vi "DriverCameraWindow.vi"() -> ()   [LabVIEW 2025]
uses:
  DashBoardGlobals.vi
panel:
  out "Camera Perf":string
  in  "Camera Settings":T1={"Frame Rate"=30, "Compression"=30, "Size"=1, "DB Camera Config"=FALSE} {"Frame Rate" scale=1.0..30.0; "Compression" scale=100.0..-1.0; "Size" items=["640x480", "640x360", "320x240", "320x180", "160x120", "160x90"]}
  out "Image Message":string="Timeout in Camera Communications"
  out "Camera Image":T2(plugin-control)
  in  "Camera Name":string(combo)="No Camera Selection"
  # "HW"
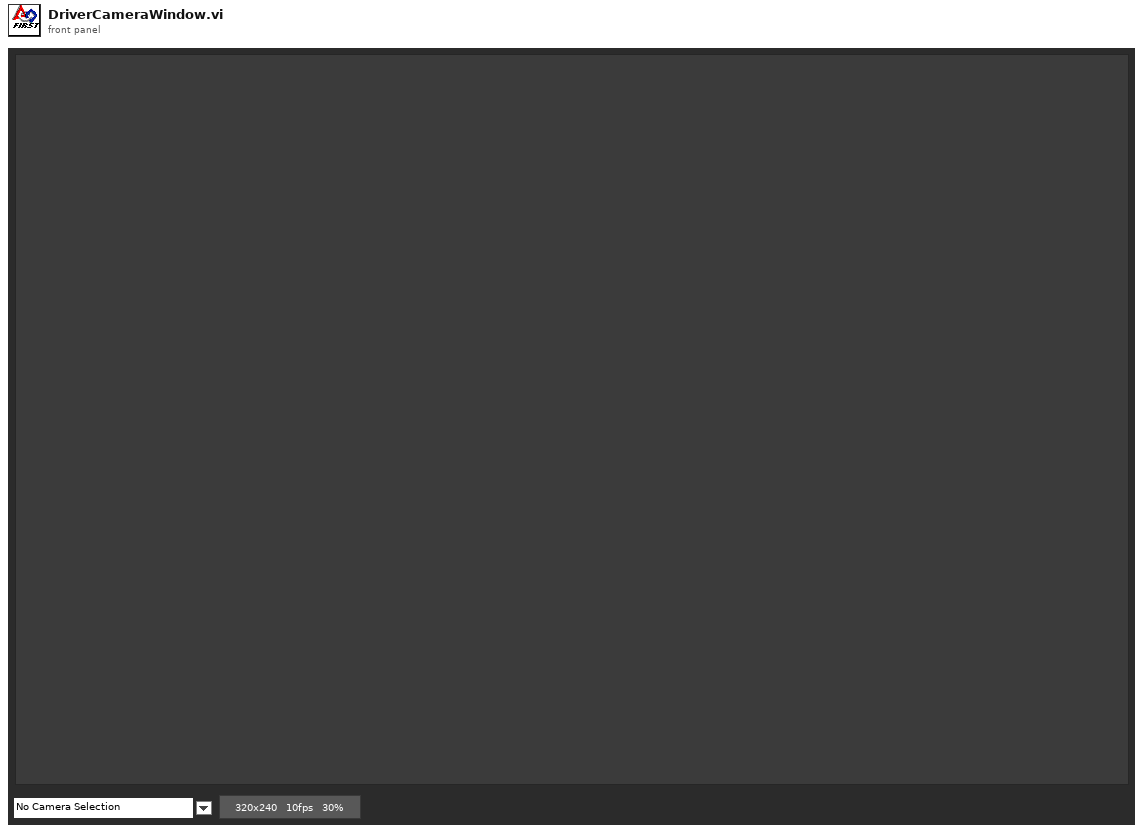
[diagram p1: front panel]
types:
  T1 = cluster{"Frame Rate":i32, "Compression":i32, "Size":u16, "DB Camera Config":bool}
  T2 = typedef "IMAQ Image.ctl" = refnum<image>
  T3 = cluster{"Save Path":path, "Interval (s)":dbl, "Keep":i32}
  T4 = typedef "Image Type" = u32
  T5 = cluster{"Global Rectangle":i32[], "Contours":cluster{"Contour Type":u32, "ROI Type":u32, "Points":i32[]}[]}
  T6 = cluster{"Camera Name":string, string, "Saved DB Images Info":cluster{"Save Path":path, "Interval (s)":dbl, "Keep":i32}}
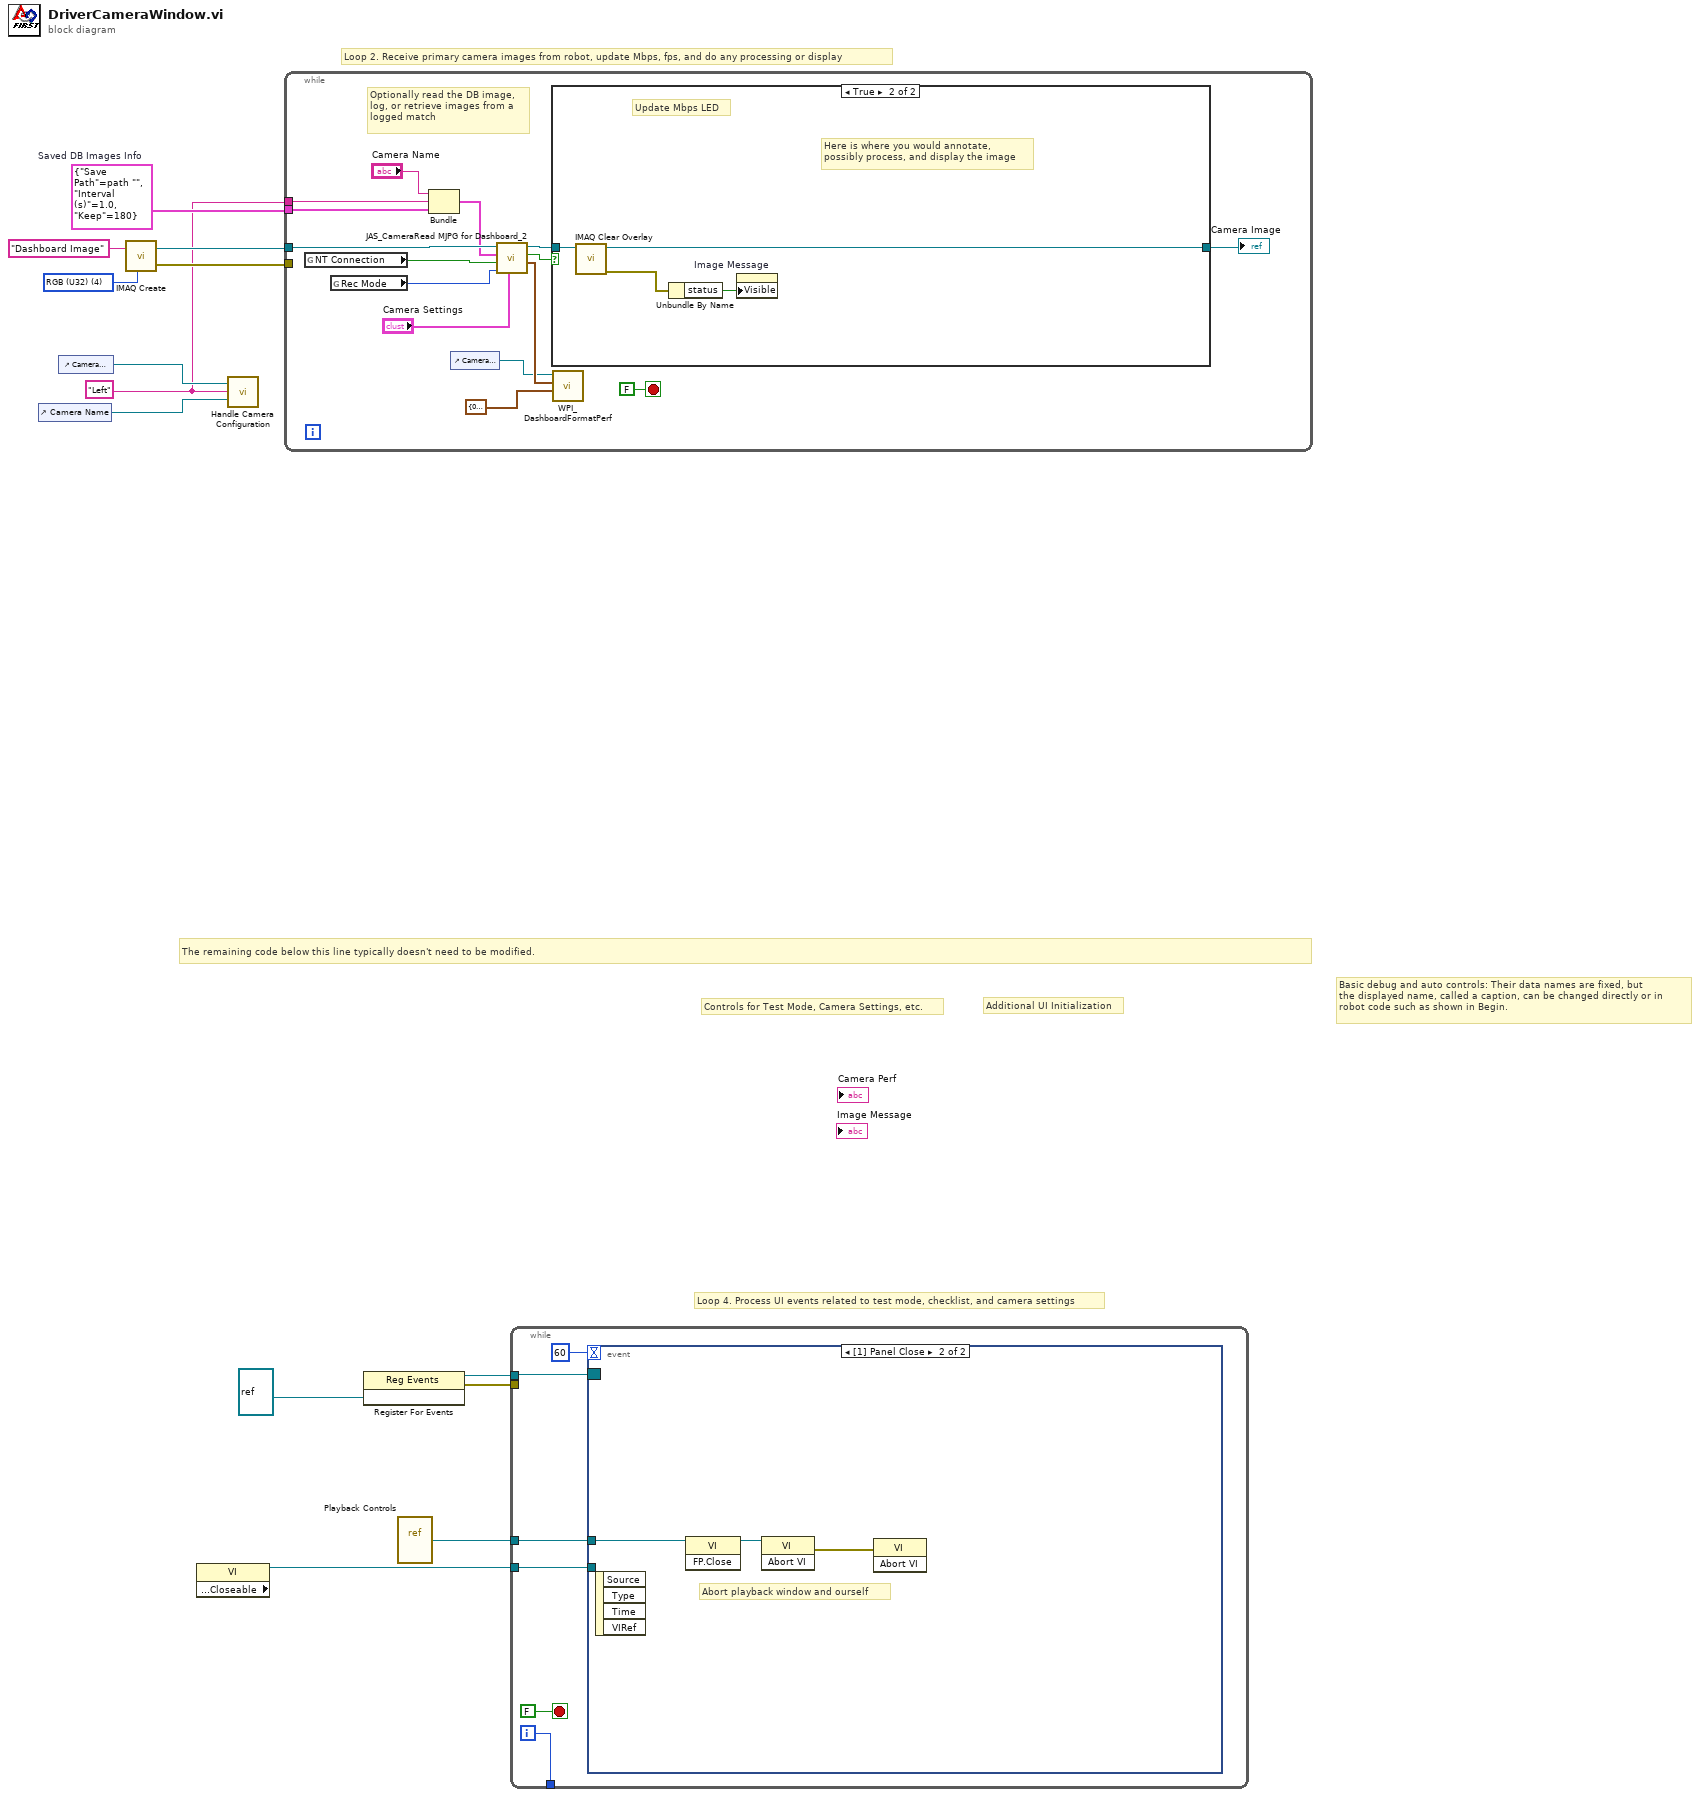
[diagram p0: block diagram]
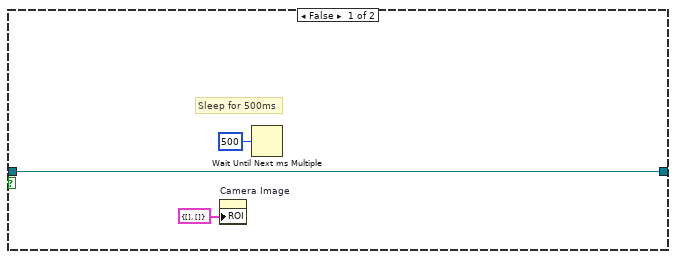
[diagram p2: hidden frame]
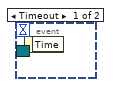
[diagram p3: hidden frame]
diagram:
  w2 = T3 {"Save Path"=path "", "Interval (s)"=1.0, "Keep"=180}  # Saved DB Images Info
  w1 = "Left"
  w13 = T4 4 items=["Grayscale (U8)", "Grayscale (I16)", "Grayscale (SGL)", "Complex (CSG)", "RGB (U32)", "HSL (U32)", "RGB (U64)"] ("Image Type")
  # "Basic debug and auto controls: Their data names are fixed, but\nthe displayed name, called a caption, can be changed directly or in\nrobot code such as shown in Begin."
  # "Controls for Test Mode, Camera Settings, etc."
  # "Additional UI Initialization"
  # "The remaining code below this line typically doesn't need to be modified."
  # "Loop 4. Process UI events related to test mode, checklist, and camera settings"
  # "Loop 2. Receive primary camera images from robot, update Mbps, fps, and do any processing or display"
  n1 = control-ref of="Camera Name"() -> (w3:refnum<vi>)
  n2 = control-ref of="Camera Settings"() -> (w4:refnum<vi>)
  n3 = call "IMAQ Create"("Image Name"="Dashboard Image", "Image Type"=w13) -> ("New Image"=w11:T2, "error out"=w10:errorcluster)  [unwired: 2 in, 1 out]
  n4 = property class="VI" props=["Front Panel.Closeable"]() -> (reference out=w5:refnum<vi>)  [unwired: 2 in, 2 out]
  n5 = call "Handle Camera Configuration.vi"("CameraNameRef"=w3, "Display Name"=w1, "ClusterRef"=w4) -> ()  [unwired: 9 in]
  n6 = while {
    tunnel: w11 -> [w27]
    tunnel: w10 -> [_]
    tunnel: w2 -> [w22]
    tunnel: w1 -> [w19]
    stop <- FALSE stop-if-true
    # "Optionally read the DB image,\nlog, or retrieve images from a\nlogged match"
    n7 = global read "DashBoardGlobals.vi" "NT Connection"() -> (w16:bool)
    n8 = global read "DashBoardGlobals.vi" "Rec Mode"() -> (w14:enum32{"Stop", "Record", "Playback"})
    n9 = Bundle("Camera Name"="Camera Name", w19, "Saved DB Images Info"=w22) -> (w21:T6)  [unwired: 1 in]
    n10 = control-ref of="Camera Perf"() -> (w17:refnum<vi>)
    n11 = call "JAS_CameraRead MJPG for Dashboard_2.vi"("Camera Settings"="Camera Settings", "Rec Mode"=w14, "NT Connection"=w16, "Capture Info"=w21, "Image in"=w27) -> ("perf info"=w18:cluster{"Bandwidth (Mbps)":dbl, "fps":dbl}, "Active"=w25:bool, "Image\\ out"=w26:T2)  [unwired: 4 in]
    n12 = case shown="True" w25 {
      tunnel: w26 -> [w30 w33]
      tunnel: [w30 w32] -> w23
      frame False {
        # "Sleep for 500ms"
        n13 = property on="Camera Image" class="ImageControl"("ROI"=T5 {"Global Rectangle"=[], "Contours"=[]}) -> ()  [unwired: 2 in, 2 out]
        n14 = Wait Until Next ms Multiple(millisecond multiple=u32 500) -> ()  [unwired: 1 out]
      }
      frame True {
        # "Here is where you would annotate,\npossibly process, and display the image"
        # "Update Mbps LED"
        n15 = call "IMAQ Clear Overlay"("Image"=w33) -> ("error out"=w34:errorcluster, "Image Out"=w32:T2)  [unwired: 2 in, 7 out]
        n16 = Unbundle By Name(w34) -> ("status"=w35:bool)
        n17 = property on="Image Message" class="Str"("Visible"=w35) -> ()  [unwired: 2 in, 2 out]
      }
    }
    "Camera Image" <- w23
    n18 = call <vilib>:"WPI_DashboardFormatPerf.vi"("Right Camera Perf"=cluster{"Bandwidth (Mbps)":dbl, "FPS":dbl} {"Bandwidth (Mbps)"=0.0, "FPS"=0.0}, "Performance"=w18, "String in"=w17) -> ()  [unwired: 9 in]
  }
  n19 = register-events(refnum<vi> refnum) -> (reference out=w8:refnum<event-registration>, error out=w7:errorcluster)  [unwired: 2 in]
  n20 = vi-ref "Playback Controls.vi"() -> (w9:refnum<vi>)
  n21 = while {
    tunnel: [w39] -> _
    tunnel: w9 -> [w38]
    tunnel: w8 -> [w37]
    tunnel: w7 -> [_]
    tunnel: w5 -> [w36]
    i -> [w39]
    stop <- FALSE stop-if-true
    n22 = event shown="[1] Panel Close" {
      selector: w37 -> [_ _]
      dyn-events: _ -> [_ _]
      timeout: u32 60 ("milliseconds to wait") -> [_ _]
      tunnel: w38 -> [_ w44]
      tunnel: w36 -> [_ _]
      event Timeout {
        n23 = event-data() -> ()  [unwired: 1 in, 1 out]
      }
      event Panel Close {
        # "Abort playback window and ourself"
        n24 = event-data() -> ()  [unwired: 1 in, 4 out]
        n25 = invoke class="VI" method="FP.Close"(reference=w44) -> (reference out=w43:refnum<vi>)  [unwired: 2 in, 2 out]
        n26 = invoke class="VI" method="Abort VI"(reference=w43) -> (error out=w42:errorcluster)  [unwired: 2 in, 2 out]
        n27 = invoke class="VI" method="Abort VI"(error in=w42) -> ()  [unwired: 2 in, 3 out]
      }
    }
  }
